vi "Flattened Call Chain.vi"() -> (1 "Flattened Call Chain":string)   [LabVIEW 2020]
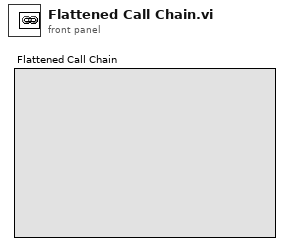
[diagram p1: front panel]
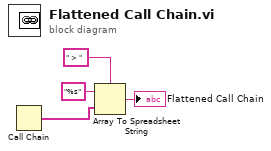
[diagram p0: block diagram]
diagram:
  n1 = Call Chain() -> (call chain=w4:string[])
  n2 = Array To Spreadsheet String(delimiter (Tab)=" > ", array=w4, 3:"%s" ("format string")) -> (spreadsheet string=→"Flattened Call Chain":string)
